vi "Snake Change Direction.vi"(8 "error in (no error)":errorcluster, 10 "Direction":T1, 11 "Snake in":refnum<class "Snake.lvclass">) -> (0 "error out":errorcluster, 3 "Snake out":refnum<class "Snake.lvclass">)   [LabVIEW 2020, in "Snake.lvclass"]
uses:
  Snake.lvclass
  Direction STYP.ctl
  Snake.lvclass/Snake.ctl
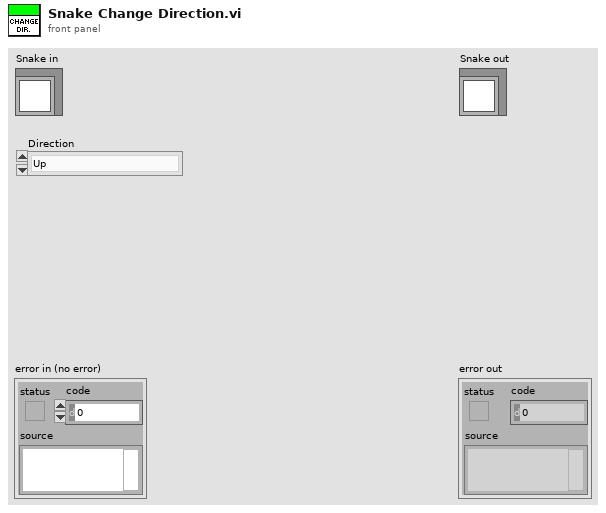
[diagram p1: front panel]
types:
  T1 = typedef "Direction STYP.ctl" = enum16{"Up", "Down", "Left", "Right"}
  T2 = typedef "Snake.lvclass/Snake Segment STYP.ctl" = cluster{"Location":cluster{"x":u32, "y":u32}, "Direction":T1}
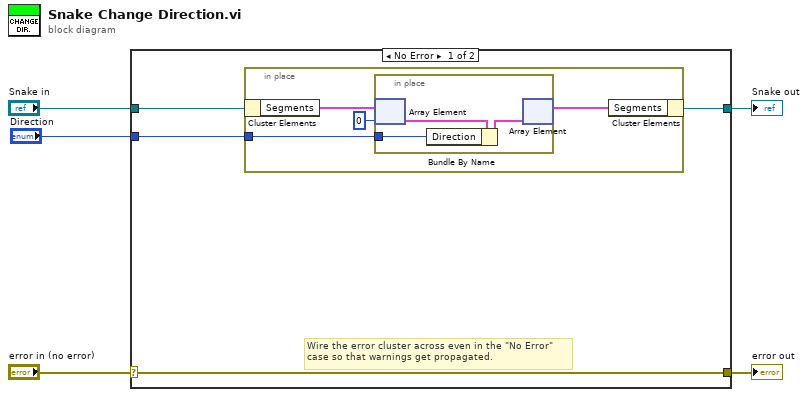
[diagram p0: block diagram]
diagram:
  n1 = case shown="No Error" "error in (no error)" {
    selector: "error in (no error)" -> [w8 w18]
    tunnel: [w8 w18] -> w4
    tunnel: [w7 w17] -> w2
    tunnel: "Snake in" -> [w9 w17]
    tunnel: "Direction" -> [w6 _]
    frame No Error {
      # "Wire the error cluster across even in the \"No Error\"\ncase so that warnings get propagated."
      n2 = in-place {
        in-place-border: w6 -> [w11]
        n3 = in-place-cluster #1(w9) -> ("Segments"=w13:T2[])
        n4 = in-place {
          in-place-border: w11 -> [w14]
          n5 = in-place-array #2(w13, 0) -> (w16:T2)
          n6 = Bundle By Name(cluster=w16, "Direction"=w14) -> (w15:T2)
          n7 = in-place-array #2(w15) -> (w12:T2[])  [unwired: 1 out]
        }
        n8 = in-place-cluster #1("Segments"=w12) -> (w7:refnum<class "Snake.lvclass">)
      }
    }
    frame Error {
    }
  }
  "error out" <- w4
  "Snake out" <- w2
